vi "Resize List.vi"(8 "error in (no error)":errorcluster caption="错误输入（无错误）", 10 "Panel Width":i16, 11 "List":refnum<vi>) -> (0 "error out":errorcluster caption="错误输出", 3 "List out":refnum<vi>)   [LabVIEW 2011, in "CAN FD.lvlib"]
uses:
  CAN FD.lvlib
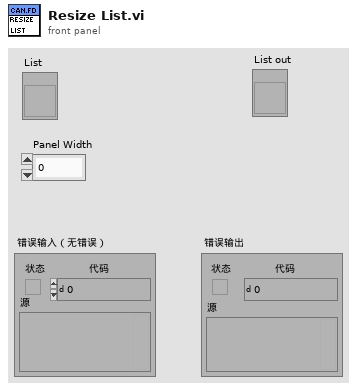
[diagram p1: front panel]
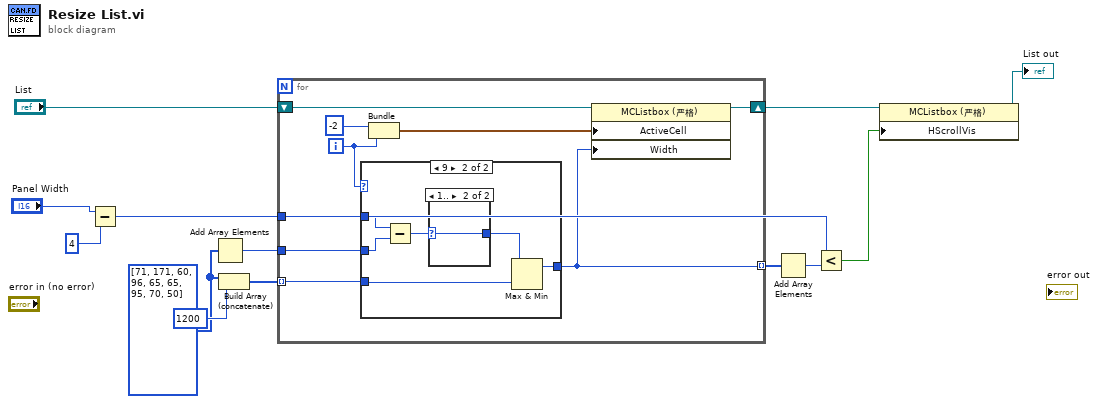
[diagram p0: block diagram]
diagram:
  w1 = u32[] [71, 171, 60, 96, 65, 65, 95, 70, 50] ("数组")
  n1 = Subtract(x="Panel Width", y=i16 4) -> (x-y=w2:i16)
  n2 = Add Array Elements(numeric array=w1) -> (sum=w11:u32)
  n3 = Build Array (concatenate)(w1, 1200 ("Width")) -> (w12:u32[])
  n4 = for {
    tunnel: w12 -> [w18] mode=indexing
    tunnel: w2 -> [w16]
    tunnel: w11 -> [w17]
    tunnel: [w15] -> w10 mode=indexing
    shift-right: [w14] -> w7
    shift-left: "List" -> [w22]
    i -> [w19]
    n5 = case shown="9" w19 {
      tunnel: w18 -> [w23 w26]
      tunnel: [w23 w24] -> w15
      tunnel: w17 -> [_ w28]
      tunnel: w16 -> [_ w29]
      frame 0, Default {
      }
      frame 9 {
        n6 = Subtract(x=w29, y=w28) -> (x-y=w27:u32)
        n7 = case shown="1.." w27 {
          selector: w27 -> [_ w30]
          tunnel: [_ w30] -> w25
          frame 0, Default {
          }
          frame 1.. {
          }
        }
        n8 = Max & Min(x=w25, y=w26) -> (max(x,y)=w24:u32)  [unwired: 1 out]
      }
    }
    n9 = Bundle(-2, w19) -> (w20:cluster{i32, i32})  [unwired: 1 in]
    n10 = property class="MCListbox (严格)"(reference=w22, "ActiveCell"=w20, "Width"=w15) -> (reference out=w14:refnum<vi>)  [unwired: 1 in, 1 out]
  }
  n11 = Add Array Elements(numeric array=w10) -> (sum=w9:u32)
  n12 = Less?(x=w2, y=w9) -> (x < y?=w6:bool)
  n13 = property class="MCListbox (严格)"(reference=w7, "HScrollVis"=w6) -> (reference out=→"List out":refnum<vi>)  [unwired: 1 in, 1 out]
